vi "ProcessHandshakeRequest.vi"(8 "error in (no error)":errorcluster, 11 "HTTP Headers":string) -> (0 "error out":errorcluster, 1 "Sec-WebSocket-Key":string, 2 "Path":string, 3 "Is Websocket Request?":bool, 4 "Headers Out":variant, 5 "Host":string, 6 "Header Array":cluster{"Name":string, "Value":string}[](array[cluster]))   [LabVIEW 2015, in "WebSockets.lvlib"]
doc: "WebSockets API 1.3.0.13\nSam Sharp - Intelligent Energy\nCopyright (c) 2015, Intelligent Energy"
uses:
  WebSockets.lvlib
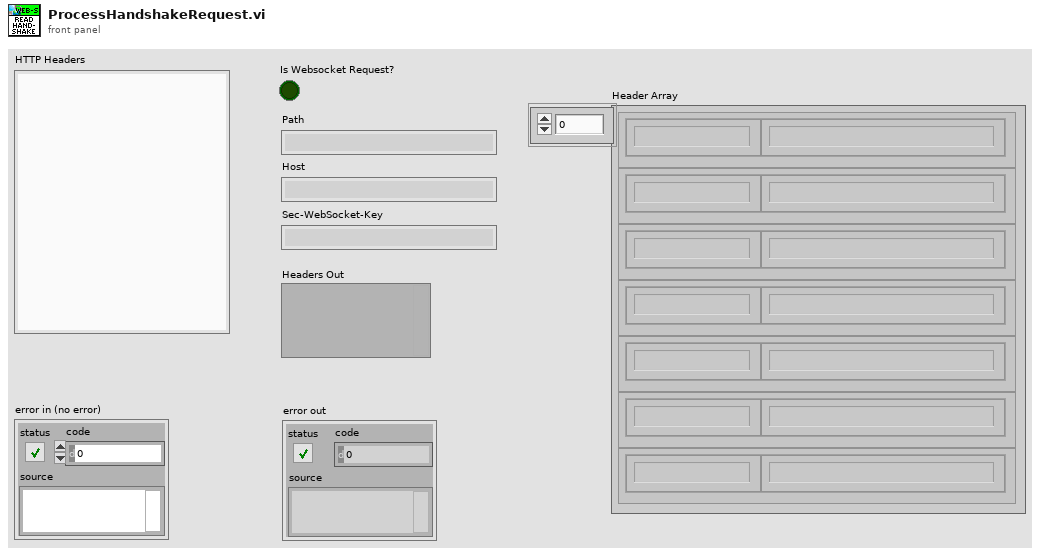
[diagram p1: front panel]
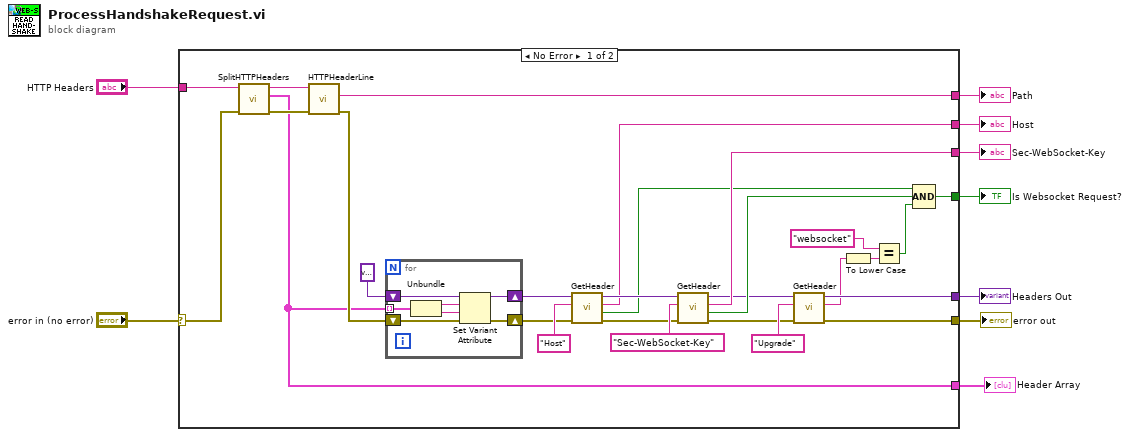
[diagram p0: block diagram]
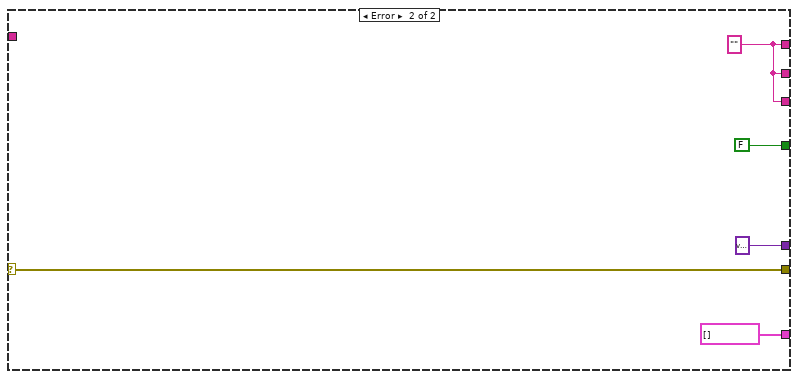
[diagram p2: hidden frame]
diagram:
  n1 = case shown="No Error" "error in (no error)" {
    selector: "error in (no error)" -> [w19 w49]
    tunnel: "HTTP Headers" -> [w37 _]
    tunnel: [w34 w47] -> w8
    tunnel: [w30 w47] -> w7
    tunnel: [w28 w47] -> w6
    tunnel: [w24 variant ("Headers Out")] -> w5
    tunnel: [w20 FALSE] -> w4
    tunnel: [w15 w49] -> w2
    tunnel: [w10 cluster{"Name":string, "Value":string}[] [] ("Header Array")] -> w1
    frame No Error {
      n2 = call "SplitHTTPHeaders.vi"("error in (no error)"=w19, "HTTP Header String"=w37) -> ("error out"=w18:errorcluster, "Header Array"=w10:cluster{"Name":string, "Value":string}[], "HTTP Request"=w36:string)  [unwired: 3 in]
      n3 = call "HTTPHeaderLine.vi"("error in (no error)"=w18, "HTTP Request Line"=w36) -> ("error out"=w13:errorcluster, "Request URI"=w34:string)  [unwired: 2 in, 2 out]
      n4 = for {
        tunnel: w10 -> [w44] mode=indexing
        shift-right: [w42] -> w33
        shift-left: variant -> [w43]
        shift-right: [w41] -> w14
        shift-left: w13 -> [w40]
        n5 = Unbundle(w44) -> ("Name"=w39:string, "Value"=w38:string)
        n6 = Set Variant Attribute(Variant=w43, name=w39, value=w38, error in=w40) -> (Variant out=w42:variant, error out=w41:errorcluster)  [unwired: 1 out]
      }
      n7 = call "GetHeader.vi"("error in (no error)"=w14, "Name"="Host" ("name"), "Headers In"=w33) -> ("error out"=w17:errorcluster, "Found?"=w27:bool, "Data"=w30:string, "Headers Out"=w31:variant)  [unwired: 1 in]
      n8 = call "GetHeader.vi"("error in (no error)"=w17, "Name"="Sec-WebSocket-Key", "Headers In"=w31) -> ("error out"=w16:errorcluster, "Found?"=w26:bool, "Data"=w28:string, "Headers Out"=w25:variant)  [unwired: 1 in]
      n9 = call "GetHeader.vi"("error in (no error)"=w16, "Name"="Upgrade", "Headers In"=w25) -> ("error out"=w15:errorcluster, "Data"=w12:string, "Headers Out"=w24:variant)  [unwired: 1 in, 1 out]
      n10 = To Lower Case(string=w12) -> (all lower case string=w11:string)
      n11 = Equal?(x="websocket", y=w11) -> (x = y?=w21:bool)
      n12 = Compound Arithmetic op=AND(w27, w26, w21) -> (w20:bool)
    }
    frame Error {
      w47 = "" ("Request URI")
    }
  }
  "Host" <- w7
  "Path" <- w8
  "Sec-WebSocket-Key" <- w6
  "Is Websocket Request?" <- w4
  "Headers Out" <- w5
  "error out" <- w2
  "Header Array" <- w1
